vi "loadDataNodeBegin.vi"(8 "error in (no error)":errorcluster, 10 "XML Refnum in":refnum<file>, 11 "xceDataNode in":refnum<class "xceDataNode.lvclass">) -> (0 "error out":errorcluster, 2 "XML Refnum out":refnum<file>, 3 "xceDataNode out":refnum<class "xceDataNode.lvclass">)   [LabVIEW 2013, in "xceDataNode.lvclass"]
doc: "Part of the file loading process. Occurs at the beginning of a node being loaded. Loads the common xceDataNode data name and description."
uses:
  xceDataNode.lvclass
  xceDataNode.lvclass/xceDataNode.ctl
  xceNode/xceNode.lvclass
  XML Parser/XML Parser.lvclass
panel:
  out "Token Found":bool
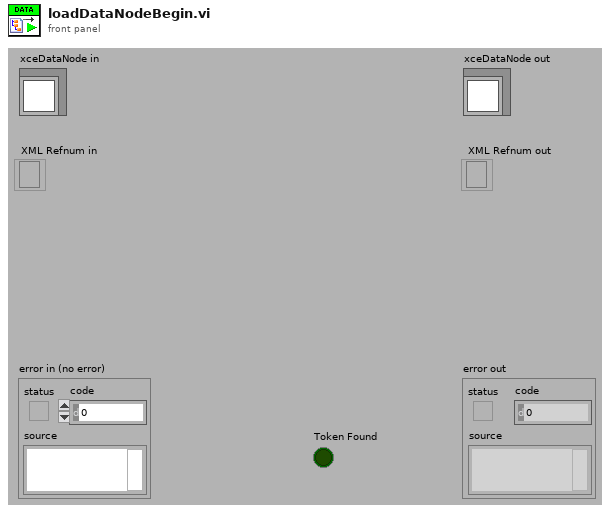
[diagram p1: front panel]
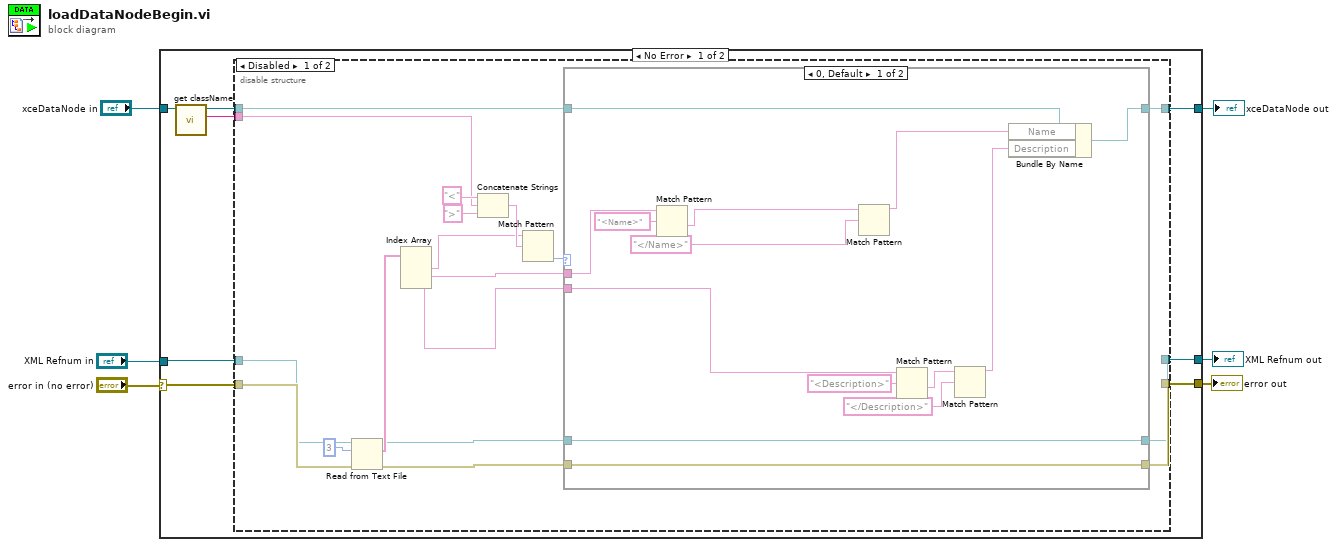
[diagram p0: block diagram]
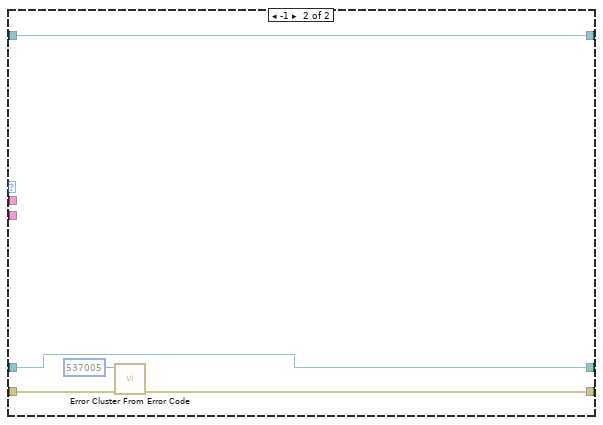
[diagram p2: hidden frame]
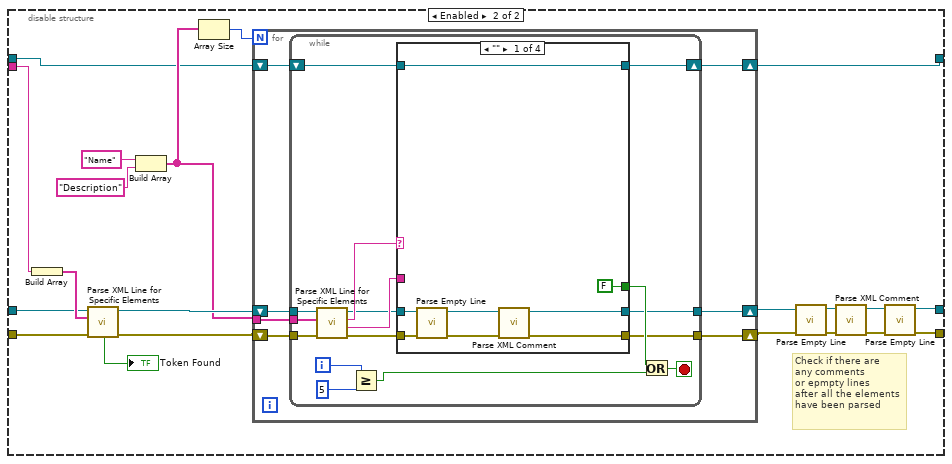
[diagram p3: hidden frame]
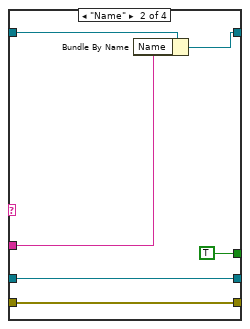
[diagram p4: hidden frame]
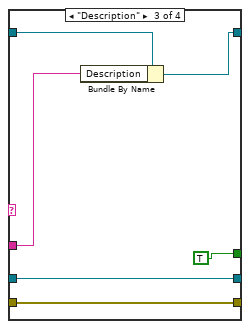
[diagram p5: hidden frame]
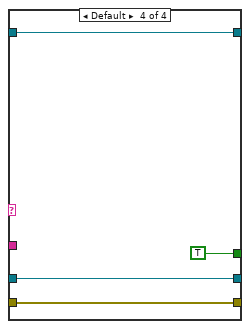
[diagram p6: hidden frame]
diagram:
  n1 = case shown="No Error" "error in (no error)" {
    selector: "error in (no error)" -> [w14 w122]
    tunnel: [w10 w122] -> w5
    tunnel: [w7 w121] -> w3
    tunnel: "xceDataNode in" -> [w12 w121]
    tunnel: "XML Refnum in" -> [w13 w120]
    tunnel: [w8 w120] -> w1
    frame No Error {
      n2 = call "get className.vi"("xceNode in"=w12) -> ("Class name"=w11:string, "xceNode out"=w9:refnum<class "xceDataNode.lvclass">)  [unwired: 8 in, 1 out]
      n3 = disable-structure shown="Disabled" {
        disable-tunnel: w14 -> [w32 w55]
        disable-tunnel: w13 -> [w31 w56]
        disable-tunnel: w11 -> [w27 w58]
        disable-tunnel: [w21 w52] -> w10
        disable-tunnel: w9 -> [w20 w57]
        disable-tunnel: [w16 w53] -> w8
        disable-tunnel: [w15 w54] -> w7
        frame Disabled {
          n4 = Read from Text File(file (use dialog)=w31, count=3, error in=w32) -> (refnum out=w17:refnum<file>, text=w29:string[], error out=w23:errorcluster)  [unwired: 1 in, 1 out]
          n5 = Index Array(array=w29) -> (element #1=w24:string, element #2=w19:string, element #3=w18:string)  [unwired: 3 in]
          n6 = Concatenate Strings("<", w27, ">" ("string")) -> (w25:string)
          n7 = Match Pattern(string=w24, regular expression=w25) -> (offset past match=w22:i32)  [unwired: 1 in, 3 out]
          n8 = case shown="0, Default" w22 {
            tunnel: w23 -> [w46 w51]
            tunnel: [w46 w50] -> w21
            tunnel: w20 -> [w44 w47]
            tunnel: w19 -> [w42 _]
            tunnel: w18 -> [w34 _]
            tunnel: w17 -> [w45 w48]
            tunnel: [w45 w48] -> w16
            tunnel: [w43 w47] -> w15
            frame 0, Default {
              n9 = Match Pattern(string=w42, regular expression="<Name>") -> (after substring=w40:string)  [unwired: 1 in, 3 out]
              n10 = Match Pattern(string=w40, regular expression="</Name>") -> (before substring=w38:string)  [unwired: 1 in, 3 out]
              n11 = Match Pattern(string=w34, regular expression="<Description>") -> (after substring=w36:string)  [unwired: 1 in, 3 out]
              n12 = Match Pattern(string=w36, regular expression="</Description>") -> (before substring=w33:string)  [unwired: 1 in, 3 out]
              n13 = Bundle By Name(cluster=w44, "Name"=w38, "Description"=w33) -> (w43:refnum<class "xceDataNode.lvclass">)
            }
            frame -1 {
              n14 = call <vilib>:"Error Cluster From Error Code.vi"("error in (no error)"=w51, "error code (0)"=537005) -> ("error out"=w50:errorcluster)  [unwired: 7 in]
            }
          }
        }
        frame Enabled {
          # "Check if there are\nany comments \nor epmpty lines\nafter all the elements\nhave been parsed"
          n15 = Build Array(w58) -> (w69:string[])
          n16 = call "Parse XML Line for Specific Elements.vi"("error in (no error)"=w55, "Elements"=w69, "XML Refnum in"=w56) -> ("error out"=w70:errorcluster, "XML Refnum out"=w71:refnum<file>, "Element Found"=→"Token Found":bool)  [unwired: 4 in, 2 out]
          n17 = Build Array("Name" ("regular expression"), "Description" ("regular expression")) -> (w61:string[])
          n18 = Array Size(array=w61) -> (size(s)=w62:i32)
          n19 = for {
            N: w62 -> [_]
            tunnel: w61 -> [w79]
            shift-right: [w74] -> w54
            shift-left: w57 -> [w76]
            shift-right: [w75] -> w67
            shift-left: w71 -> [w78]
            shift-right: [w73] -> w68
            shift-left: w70 -> [w77]
            n20 = while {
              tunnel: w79 -> [w95]
              tunnel: w78 -> [w94]
              tunnel: w77 -> [w93]
              shift-right: [w88] -> w74
              shift-left: w76 -> [w90]
              tunnel: [w80] -> w75
              tunnel: [w81] -> w73
              i -> [w92]
              stop <- w85 stop-if-true
              n21 = call "Parse XML Line for Specific Elements.vi"("error in (no error)"=w93, "Elements"=w95, "XML Refnum in"=w94) -> ("error out"=w82:errorcluster, "Value"=w84:string, "Element Name"=w89:string, "XML Refnum out"=w83:refnum<file>)  [unwired: 4 in, 1 out]
              n22 = Greater Or Equal?(x=w92, y=5) -> (x >= y?=w86:bool)
              n23 = case shown="\"\"" w89 {
                tunnel: w90 -> [w103 w109 w115 w119]
                tunnel: [w103 w108 w114 w119] -> w88
                tunnel: [FALSE TRUE TRUE TRUE] -> w87
                tunnel: w84 -> [_ w104 w113 _]
                tunnel: w83 -> [w102 w106 w111 w117]
                tunnel: w82 -> [w101 w105 w110 w116]
                tunnel: [w98 w105 w110 w116] -> w81
                tunnel: [w97 w106 w111 w117] -> w80
                frame "" {
                  n24 = call "Parse Empty Line.vi"("error in (no error)"=w101, "XML Refnum in"=w102) -> ("error out"=w99:errorcluster, "XML Refnum out"=w100:refnum<file>)  [unwired: 7 in, 1 out]
                  n25 = call "Parse XML Comment.vi"("error in (no error)"=w99, "XML Refnum in"=w100) -> ("error out"=w98:errorcluster, "XML Refnum out"=w97:refnum<file>)  [unwired: 6 in, 2 out]
                }
                frame "Name" {
                  n26 = Bundle By Name(cluster=w109, "Name"=w104) -> (w108:refnum<class "xceDataNode.lvclass">)
                }
                frame "Description" {
                  n27 = Bundle By Name(cluster=w115, "Description"=w113) -> (w114:refnum<class "xceDataNode.lvclass">)
                }
                frame Default {
                }
              }
              n28 = Or(x=w87, y=w86) -> (x .or. y?=w85:bool)
            }
          }
          n29 = call "Parse Empty Line.vi"("error in (no error)"=w68, "XML Refnum in"=w67) -> ("error out"=w64:errorcluster, "XML Refnum out"=w63:refnum<file>)  [unwired: 7 in, 1 out]
          n30 = call "Parse XML Comment.vi"("error in (no error)"=w64, "XML Refnum in"=w63) -> ("error out"=w66:errorcluster, "XML Refnum out"=w65:refnum<file>)  [unwired: 6 in, 2 out]
          n31 = call "Parse Empty Line.vi"("error in (no error)"=w66, "XML Refnum in"=w65) -> ("error out"=w52:errorcluster, "XML Refnum out"=w53:refnum<file>)  [unwired: 7 in, 1 out]
        }
      }
    }
    frame Error {
    }
  }
  "error out" <- w5
  "xceDataNode out" <- w3
  "XML Refnum out" <- w1
